vi "8channel_sEMG_main.vi"(0 "VISA resource name":refnum<visa-resource-name>="COM5", 1 "baud rate":u32=2000000, 2 "data bits":u16=8 min=5 max=8 step=1, 3 "parity":u16(ring) items=["None", "Odd", "Even", "Mark", "Space"], 4 "stop bits":u16(ring)=10 items=["1.0"=10, "1.5"=15, "2.0"=20], 7 "flow control":u16(ring) items=["None"=0, "XON/XOFF"=1, "RTS/CTS"=2, "DTR/DSR"=4]) -> ()   [LabVIEW 2023]
doc: "The Basic Serial Read and Write example performs a Serial Port Read, a Serial Port Write, or a combination of these actions. The user selects the actions (read or write) on the front panel. If both are selected, the VI will write the data first, read data, and then close the VISA session that is opened to the port. This VI will wait until the specified number of bytes is received at the port or until a termination character is read.\n\nINSTRUCTIONS:\n1) Select the serial resource and configuration parameters (baud rate, data bits, parity, stop bits, flow control).\n2) Select the operations to be performed. \n3) Connect the serial port to your device. If no device is available, perform a loopback test by doing one of the following. Short pins 2 and 3 on a RS-232 cable or short pin 4 to pin 8 and pin 5 to pin 9 on a RS-485/422 cable. \n4) Run the VI to see the data read. (The \"read string\" will match the \"string to write\" if a loopback test was performed.)\n\nNote: The parameters set for the serial port must match the parameters of the connected instrument or device. In this example, the bytes to read parameter specifies the number of bytes that the serial port reads. If there were more bytes at the port than the number specified in bytes to read, those bytes would not be read. Also, if you specify to read more bytes than the number of bytes actually read, you might receive a timeout error message.\n\nOn the block diagram, the Configure Serial Port VI sets the configuration parameters. The front panel displays the controls used to configure the basic parameters, such as baud rate, data bits, and parity. Constants configure the other parameters the user probably does not need set. After the VISA Configure Serial Port VI opens the VISA session and configures the port, the VI passes the VISA resource name to other VIs that perform operations on that VISA resource. The VISA Write function sends a command to the serial device and the VISA Read function returns data based on the command. The VISA Close function then closes the reference to the serial device. It is important to close the reference; otherwise communication through with that port through protocols other than VISA might not be possible."
uses:
  <vilib>/Instr/_visa.llb/VISA Configure Serial Port (Instr).vi
panel:
  in  "Apply":bool
  in  "Filters":T1={"Bandstop"=enum."50 x N", "Bandpass low/high"={5, 500}}
  in  "Stop program":bool
  in  "Sampling frequency":dbl=2000.0
  in  "?":T2(tab)
  in  "Plot on/off":bool
  out "EMG plots":T3
  out "Mean Frequency":dbl
  in  "Frequency on/off":bool
  out "Spectrum":dbl[](graph)
  out "?":i32(graph)=145
  in  "Channel":i32=1
  out "Channel RMS":dbl(slide) scale=0.0..1000.0
  out "Weighted sum":dbl[](array[slide]) scale=-1000.0..2000.0
  in  "Index of Command to delete":i8
  in  "Delete Command":bool
  in  "Add Command":bool
  in  "RMS sample length":i32=1000
  in  "RMS on/off":bool
  out "RMS data":T4 {"RMS 8" scale=0.0..100.0; "RMS 7" scale=0.0..100.0; "RMS 6" scale=0.0..100.0; "RMS 5" scale=0.0..100.0; "RMS 4" scale=0.0..2000.0; "RMS 3" scale=0.0..2000.0; "RMS 2" scale=0.0..2000.0; "RMS 1" scale=0.0..2000.0}
  in  "Command To Add":T5={"Threshold"=1000.0, "Weights for new action"={"W 1"=0.0, "W 2"=0.0, "W 3"=0.0, "W 4"=0.0, "W 5"=0.0, "W 6"=0.0, "W 7"=0.0, "W 8"=0.0}, "Virtual Key"=87} {"Weights for new action"."W 8" scale=-10.0..10.0; "Weights for new action"."W 7" scale=-10.0..10.0; "Weights for new action"."W 6" scale=-10.0..10.0; "Weights for new action"."W 5" scale=-10.0..10.0; "Weights for new action"."W 4" scale=-10.0..10.0; "Weights for new action"."W 3" scale=-10.0..10.0; "Weights for new action"."W 2" scale=-10.0..10.0; "Weights for new action"."W 1" scale=-10.0..10.0}
  out "Array of commands":T6(array[cluster]) {"Weights for action"."W 8" scale=-10.0..10.0; "Weights for action"."W 7" scale=-10.0..10.0; "Weights for action"."W 6" scale=-10.0..10.0; "Weights for action"."W 5" scale=-10.0..10.0; "Weights for action"."W 4" scale=-10.0..10.0; "Weights for action"."W 3" scale=-10.0..10.0; "Weights for action"."W 2" scale=-10.0..10.0; "Weights for action"."W 1" scale=-10.0..10.0}
  in  "Send key commands":bool
  in  "Apply RMS window":bool
  out "Leftover length":dbl
  out "Bytes read":dbl
  out "Leftover":string
  out "String in":string="C00000,011E2E,F8A5FE,FFFCCF,FFF7A8,FFFB31,FFFC87,FFF9B0,FFFC2D,\r\n"
  out "Stat":string="C00000"
  out "Bytes at Serial Port":u32=3929
  out "Samples per read":i32
  in  "Loop update speed":dbl=0.5 format="%#_13g"
  in  "Wait for bytes":u32=49
  out "Double data values":T7
  in  "Queue":bool=TRUE
  in  "Record":bool
  out "# elements in queue":i32
  in  "file path":path
  out "Create file":errorcluster
  out "millisecond timer value":u32 format="%<%H:%M>t"
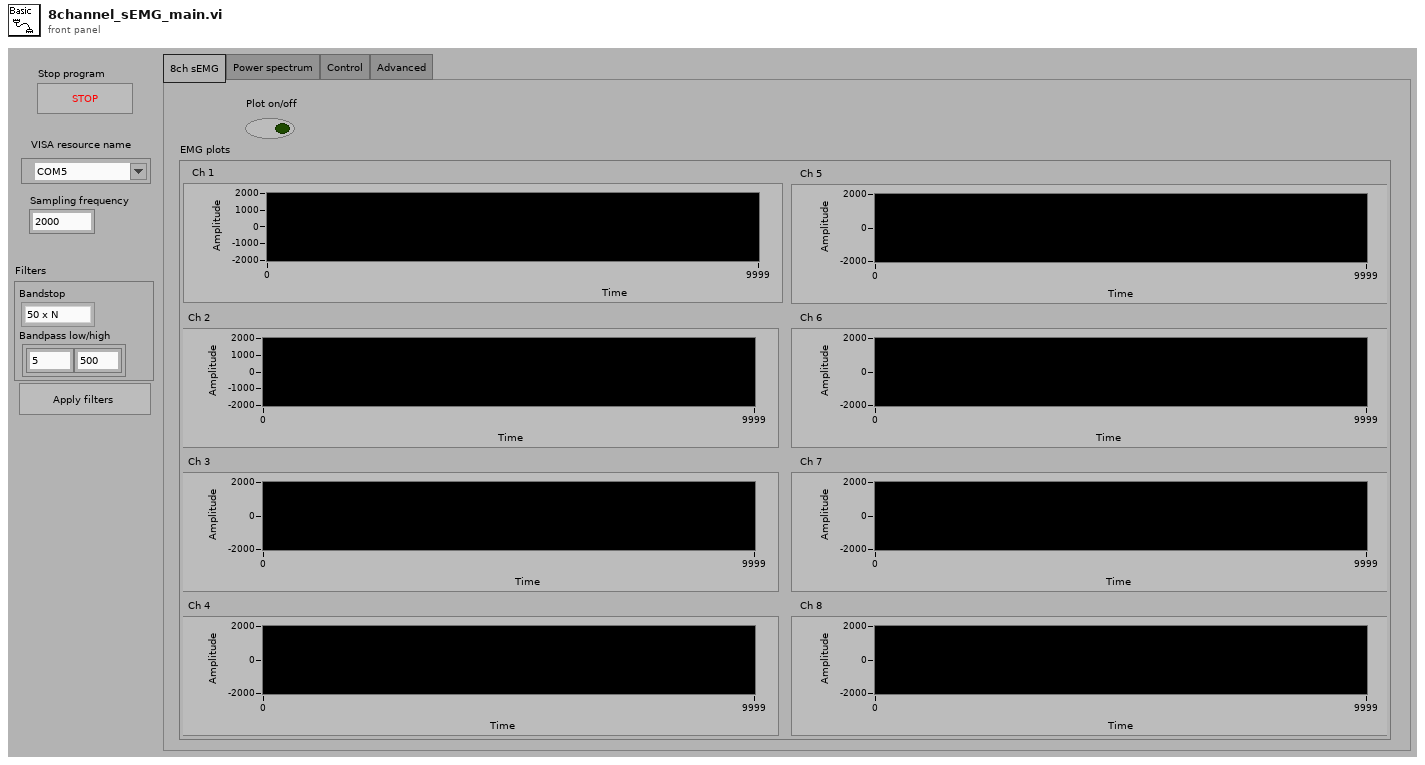
[diagram p1: front panel]
types:
  T1 = cluster{"Bandstop":enum16{"None", "50", "50 x N"}, "Bandpass low/high":cluster{i32, i32}}
  T2 = enum32{"8ch sEMG", "Power spectrum", "Control", "Advanced"}
  T3 = cluster{"Ch 1":dbl[], "Ch 2":dbl[], "Ch 3":dbl[], "Ch 4":dbl[], "Ch 5":dbl[], "Ch 6":dbl[], "Ch 7":dbl[], "Ch 8":dbl[]}
  T4 = cluster{"RMS data array[0]":dbl, "RMS data array[1]":dbl, "RMS data array[2]":dbl, "RMS data array[3]":dbl, "RMS data array[4]":dbl, "RMS data array[5]":dbl, "RMS data array[6]":dbl, "RMS data array[7]":dbl}
  T5 = cluster{"Threshold":dbl, "Weights for new action":cluster{"W 1":dbl, "W 2":dbl, "W 3":dbl, "W 4":dbl, "W 5":dbl, "W 6":dbl, "W 7":dbl, "W 8":dbl}, "Virtual Key":u8}
  T6 = cluster{"Threshold":dbl, "Weights for action":cluster{"W 1":dbl, "W 2":dbl, "W 3":dbl, "W 4":dbl, "W 5":dbl, "W 6":dbl, "W 7":dbl, "W 8":dbl}, "Virtual Key":u8}[]
  T7 = cluster{"Data in":dbl, "Data in":dbl, "Data in":dbl, "Data in":dbl, "Data in":dbl, "Data in":dbl, "Data in":dbl, "Data in":dbl}
  T8 = enum16{"open", "open or create", "create or replace", "create", "open (read-only)"}
  T9 = cluster{"[0]":dbl, "[1]":dbl, "[2]":dbl, "[3]":dbl, "[4]":dbl, "[5]":dbl, "[6]":dbl, "[7]":dbl}
  T10 = cluster{"Filtered data array":dbl[], "Filtered data array":dbl[], "Filtered data array":dbl[], "Filtered data array":dbl[], "Filtered data array":dbl[], "Filtered data array":dbl[], "Filtered data array":dbl[], "Filtered data array":dbl[]}
  T11 = cluster{"W 1":dbl, "W 2":dbl, "W 3":dbl, "W 4":dbl, "W 5":dbl, "W 6":dbl, "W 7":dbl, "W 8":dbl}
  T12 = cluster{"Threshold":dbl, "Weights for new action":cluster{"W 1":dbl, "W 2":dbl, "W 3":dbl, "W 4":dbl, "W 5":dbl, "W 6":dbl, "W 7":dbl, "W 8":dbl}, "Virtual Key":u8}[]
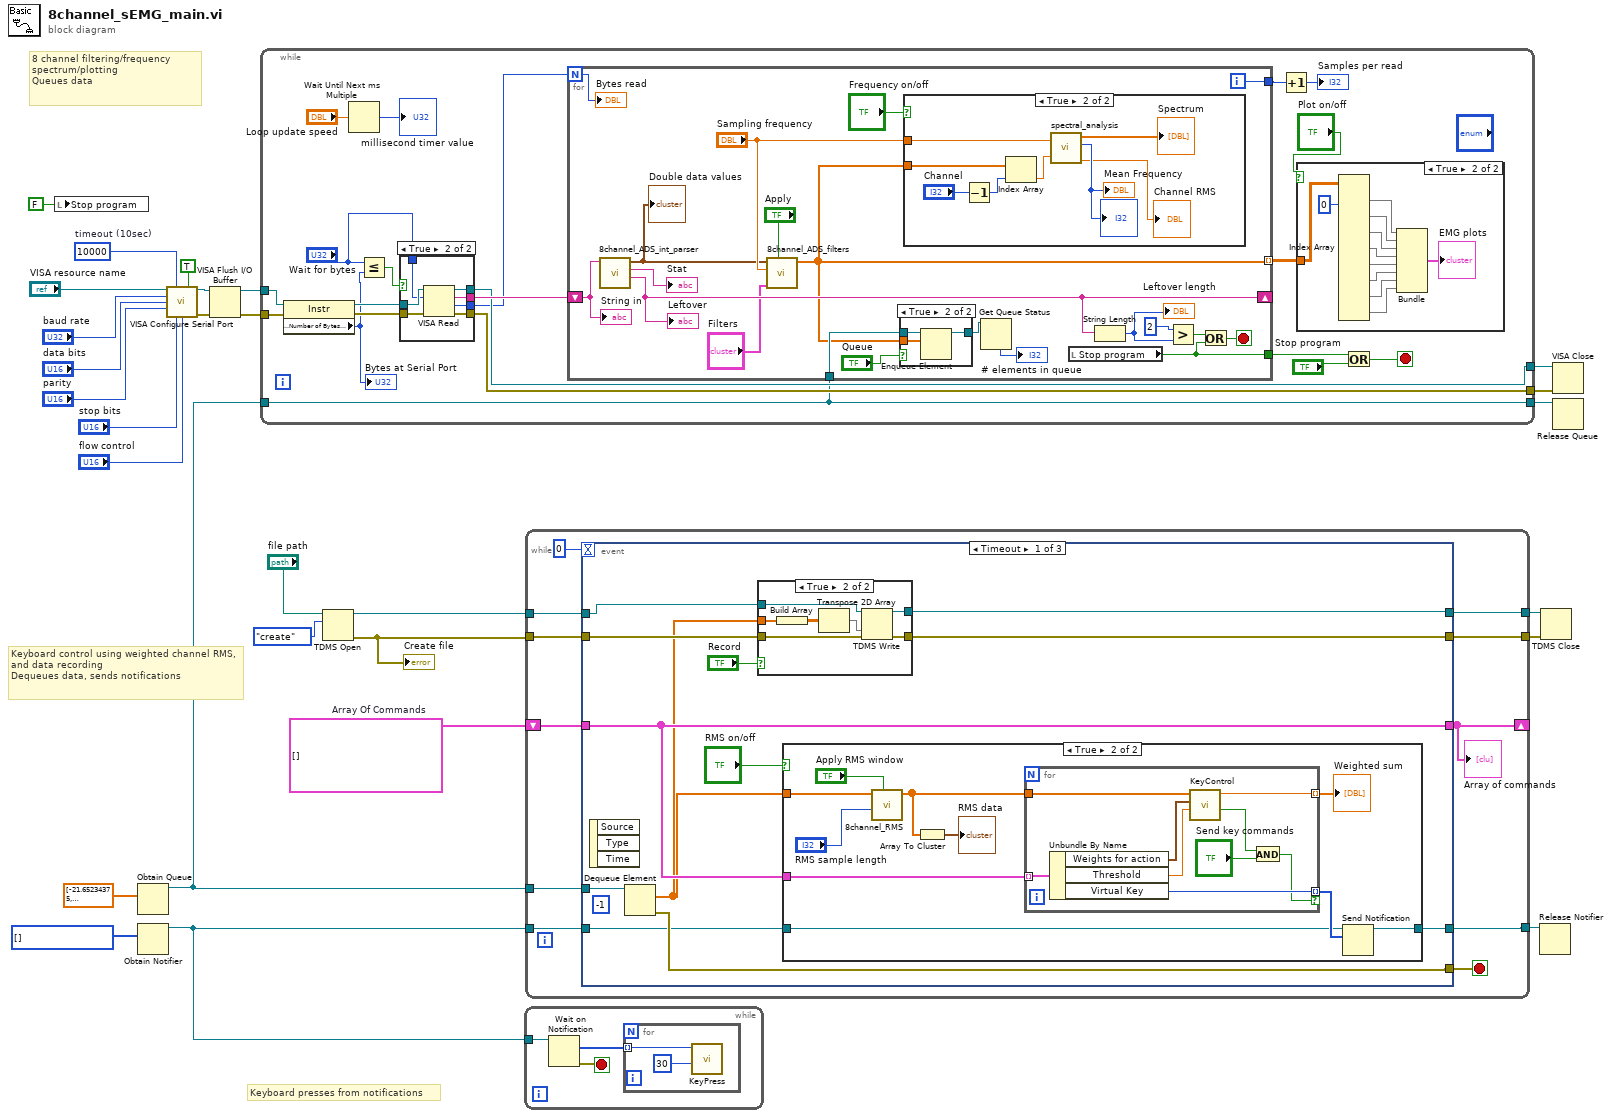
[diagram p0: block diagram]
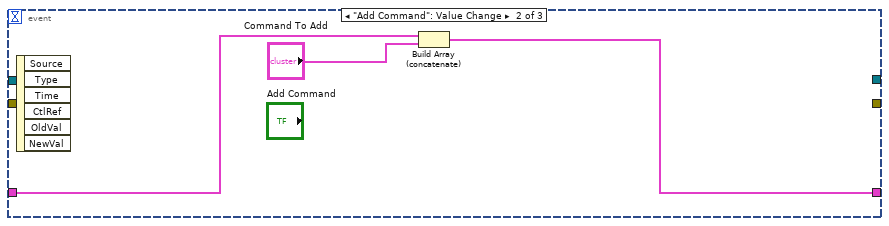
[diagram p4: hidden frame]
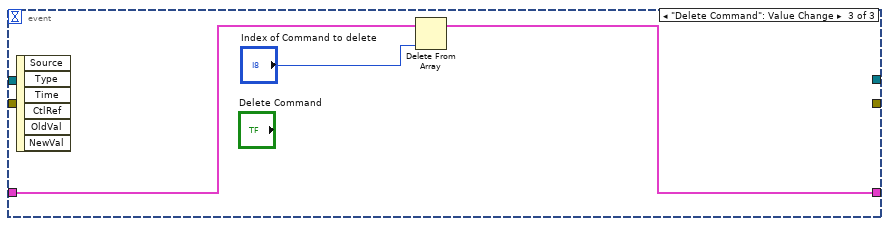
[diagram p5: hidden frame]
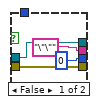
[diagram p6: hidden frame]
diagram:
  w9 = T6 []  # Array Of Commands
  w23 = u32 10000  # timeout (10sec)
  # "Keyboard presses from notifications"
  # "Keyboard control using weighted channel RMS, and data recording\nDequeues data, sends notifications"
  # "8 channel filtering/frequency spectrum/plotting\nQueues data"
  n1 = local write "Stop program"(FALSE ("stop")) -> ()
  n2 = Obtain Queue(element data type=dbl[] [-21.65234375, -13.739501953125, 40.8359375, 9.593017578125, 0.0, 0.0, 0.0, 0.0] ("Filtered data array")) -> (queue out=w14:refnum<queue>)  [unwired: 4 in, 2 out]
  n3 = Obtain Notifier(notification data type=u8[] [] ("Virtual Key 3")) -> (notifier out=w13:refnum<notifier>)  [unwired: 3 in, 2 out]
  n4 = call-poly "VISA Configure Serial Port"("VISA resource name"="VISA resource name", "timeout (10sec)"=w23, "Enable Termination\nChar (T)"=TRUE ("Enable Termination\nChar (T)"), "baud rate (9600)"="baud rate", "data bits (8)"="data bits", "parity (0:none)"="parity", "stop bits (10: 1 bit)"="stop bits", "flow control (0:none)"="flow control") -> ("VISA resource name out"=w16:refnum<visa-resource-name>, "error out"=w15:errorcluster)  [unwired: 1 in, 5 out]
  n5 = VISA Flush I/O Buffer(VISA resource name=w16, error in (no error)=w15) -> (VISA resource name out=w18:refnum<visa-resource-name>, error out=w17:errorcluster)  [unwired: 1 in]
  n6 = while {
    tunnel: [w49] -> w26
    tunnel: [w39] -> w25
    tunnel: w18 -> [w48]
    tunnel: w17 -> [w47]
    tunnel: w14 -> [w32]
    tunnel: [w32] -> w11
    stop <- w42 stop-if-true
    n7 = property class="Instr"(reference=w48, error in=w47) -> (reference out=w46:refnum<visa-resource-name>, error out=w45:errorcluster, "Serial Settings:Number of Bytes at Serial Port"=w31:u32)
    "Bytes at Serial Port" <- w31
    n8 = Wait Until Next ms Multiple(millisecond multiple="Loop update speed") -> (millisecond timer value=→"millisecond timer value":u32)
    n9 = Less Or Equal?(x="Wait for bytes", y=w31) -> (x <= y?=w33:bool)
    n10 = case shown="True" w33 {
      tunnel: [w53 w60] -> w49
      tunnel: w46 -> [w52 w59]
      tunnel: w45 -> [w53 w58]
      tunnel: ["\"\"" ("read buffer") w57] -> w44
      tunnel: [w52 w56] -> w39
      tunnel: [u32 0 ("return count") w55] -> w37
      tunnel: "Wait for bytes" -> [_ w54]
      frame False {
      }
      frame True {
        n11 = VISA Read(VISA resource name=w59, byte count=w54, error in (no error)=w58) -> (VISA resource name out=w56:refnum<visa-resource-name>, read buffer=w57:string, return count=w55:u32, error out=w60:errorcluster)
      }
    }
    n12 = for {
      N: w37 -> [w75]
      shift-right: [w84] -> _
      shift-left: w44 -> [w76]
      tunnel: [w86] -> w40
      tunnel: [w77] -> w41 mode=indexing
      tunnel: w32 -> [w82]
      tunnel: [w74] -> w35
      i -> [w74]
      stop <- w87 stop-if-true
      n13 = call "8channel_ADS_int_parser.vi"("String in"=w76) -> ("Leftover"=w84:string, "Stat"=→"Stat":string, "Data out"=w72:T9)  [unwired: 8 in]
      "Leftover" <- w84
      "Double data values" <- w72
      n14 = call "8channel_ADS_filters.vi"("Apply"="Apply", "Filters"="Filters", "Sampling frequency"="Sampling frequency", "Data in 8 ch"=w72) -> ("Filtered data array"=w77:dbl[])  [unwired: 7 in]
      n15 = case shown="True" "Queue" {
        tunnel: w82 -> [w92 w95]
        tunnel: [w92 w94] -> w81
        tunnel: w77 -> [_ w93]
        frame False {
        }
        frame True {
          n16 = Enqueue Element(queue=w95, element=w93) -> (queue out=w94:refnum<queue>)  [unwired: 2 in, 2 out]
        }
      }
      n17 = case shown="True" "Frequency on/off" {
        tunnel: "Sampling frequency" -> [_ w101]
        tunnel: w77 -> [_ w100]
        frame False {
        }
        frame True {
          n18 = Decrement(x="Channel") -> (x-1=w96:i32)
          n19 = Index Array(array=w100, index=w96) -> (element=w99:dbl)
          n20 = call "spectral_analysis.vi"("Sampling frequency"=w101, "Data"=w99) -> ("Spectrum"=→"Spectrum":dbl[], 3:→"?" →"Mean Frequency":i32, "RMS"=→"Channel RMS":dbl)  [unwired: 1 in]
        }
      }
      n21 = Get Queue Status(queue=w81) -> (# elements in queue=→"# elements in queue":i32)  [unwired: 2 in, 7 out]
      n22 = local read "Stop program"() -> (w86:bool)
      n23 = String Length(string=w84) -> (length=w90:i32)
      "Leftover length" <- w90
      n24 = Greater?(x=2, y=w90) -> (0:w89:bool)
      n25 = Or(x=w89, y=w86) -> (x .or. y?=w87:bool)
      "String in" <- w76
      "Bytes read" <- w75
    }
    n26 = Increment(x=w35) -> (x+1=→"Samples per read":i32)
    n27 = case shown="True" "Plot on/off" {
      tunnel: w41 -> [_ w71]
      frame False {
      }
      frame True {
        n28 = Index Array(array=w71, index (col) #1=0 ("index (col)")) -> (element #1=w70:dbl[], element #2=w69:dbl[], element #3=w68:dbl[], element #4=w67:dbl[], element #5=w66:dbl[], element #6=w65:dbl[], element #7=w64:dbl[], element #8=w63:dbl[])  [unwired: 15 in]
        n29 = Bundle("Filtered data array"=w70, "Filtered data array"=w69, "Filtered data array"=w68, "Filtered data array"=w67, "Filtered data array"=w66, "Filtered data array"=w65, "Filtered data array"=w64, "Filtered data array"=w63) -> (→"EMG plots":T10)  [unwired: 1 in]
      }
    }
    n30 = Or(x=w40, y="Stop program") -> (x .or. y?=w42:bool)
  }
  n31 = TDMS Open(10:T8."create" ("operation (0:open)"), 11:"file path") -> (0:w1:errorcluster, 3:w6:refnum<k34>)  [unwired: 5 in]
  "Create file" <- w1
  n32 = while {
    tunnel: w13 -> [w106]
    stop <- w105 stop-if-true
    n33 = Wait on Notification(notifier=w106) -> (notification=w104:u8[], error out=w105:errorcluster)  [unwired: 3 in, 2 out]
    n34 = for {
      tunnel: w104 -> [w107] mode=indexing
      n35 = call "KeyPress.vi"("Millis"=u32 30 ("Length of Key Press (ms)"), "Virtual Key"=w107) -> ()  [unwired: 10 in]
    }
  }
  n36 = while {
    tunnel: w14 -> [w119]
    tunnel: w13 -> [w116]
    tunnel: [w117] -> w12
    shift-right: [w113] -> _
    shift-left: w9 -> [w114]
    tunnel: w6 -> [w112]
    tunnel: [w111] -> w5
    tunnel: w1 -> [w110]
    tunnel: [w109] -> w4
    stop <- w118 stop-if-true
    n37 = event shown="[0] Timeout" {
      selector: _ -> [_ _ _]
      dyn-events: _ -> [_ _ _]
      timeout: 0 -> [_ _ _]
      tunnel: w119 -> [w131 _ _]
      tunnel: [w130 _ _] -> w118
      tunnel: [w129 _ _] -> w117
      tunnel: w116 -> [w128 _ _]
      tunnel: w114 -> [w127 w163 w166]
      tunnel: [w127 w161 w165] -> w113
      tunnel: w112 -> [w125 _ _]
      tunnel: [w124 _ _] -> w111
      tunnel: w110 -> [w123 _ _]
      tunnel: [w120 _ _] -> w109
      event Timeout {
        (unwired) -1 ("timeout in ms (-1)")
        n38 = event-data() -> ()  [unwired: 1 in, 3 out]
        n39 = Dequeue Element(queue=w131) -> (element=w122:dbl[], error out=w130:errorcluster)  [unwired: 2 in, 2 out]
        n40 = case shown="True" "Record" {
          tunnel: w125 -> [w133 w140]
          tunnel: [w133 w139] -> w124
          tunnel: w123 -> [w132 w138]
          tunnel: [w132 w137] -> w120
          tunnel: w122 -> [_ w135]
          frame False {
          }
          frame True {
            n41 = Build Array(w135) -> (w136:dbl[][])
            n42 = Transpose 2D Array(2D array=w136) -> (transposed array=w134:dbl[][])
            n43 = TDMS Write(0:w140, 9:w134, 11:w138) -> (4:w139:refnum<k34>, 15:w137:errorcluster)  [unwired: 3 in, 2 out]
          }
        }
        n44 = case shown="True" "RMS on/off" {
          tunnel: [w141 w150] -> w129
          tunnel: w128 -> [w141 w148]
          tunnel: w127 -> [_ w147]
          tunnel: w122 -> [_ w144]
          frame False {
          }
          frame True {
            n45 = call "8channel_RMS.vi"("Apply"="Apply RMS window", "sample length"="RMS sample length", "Input"=w144) -> ("RMS data array"=w143:dbl[])  [unwired: 8 in]
            n46 = Array To Cluster(array=w143) -> (cluster=→"RMS data":T4)
            n47 = for {
              tunnel: w143 -> [w156]
              tunnel: w147 -> [w160] mode=indexing
              tunnel: [w157] -> w149 mode=indexing if=w154
              tunnel: [w155] -> w146 mode=indexing
              n48 = Unbundle By Name(w160) -> ("Weights for action"=w158:T11, "Threshold"=w159:dbl, "Virtual Key"=w157:u8)
              n49 = call "KeyControl.vi"("Threshold"=w159, "Channel weights"=w158, "Input"=w156) -> ("x > y?"=w153:bool, "sum"=w155:dbl)  [unwired: 7 in]
              n50 = And(x=w153, y="Send key commands") -> (x .and. y?=w154:bool)
            }
            "Weighted sum" <- w146
            n51 = Send Notification(notification=w149, notifier=w148) -> (notifier out=w150:refnum<notifier>)  [unwired: 1 in, 1 out]
          }
        }
      }
      event "Add Command": Value Change {
        n52 = event-data() -> ()  [unwired: 1 in, 6 out]
        n53 = Build Array (concatenate)(w163, "Command To Add") -> (w161:T12)
      }
      event "Delete Command": Value Change {
        n54 = event-data() -> ()  [unwired: 1 in, 6 out]
        n55 = Delete From Array(array=w166, index="Index of Command to delete") -> (array with subset deleted=w165:T6)  [unwired: 1 in, 1 out]
      }
    }
    "Array of commands" <- w113
  }
  n56 = Release Notifier(notifier=w12) -> ()  [unwired: 2 in, 3 out]
  n57 = TDMS Close(8:w4, 11:w5) -> ()  [unwired: 2 out]
  n58 = VISA Close(VISA resource name=w25, error in (no error)=w26) -> ()  [unwired: 1 out]
  n59 = Release Queue(queue=w11) -> ()  [unwired: 2 in, 3 out]
